vi "Check new DelayFormula and Update DelaysHW.vi"(7 "Update HW?(false)":bool, 8 "error in (no error)":errorcluster, 9 "Delay Formula":string, 10 "ChnlName":string, 11 "BME_DG_System in":refnum<class "BME_DG_System.lvclass">) -> (0 "error out":errorcluster, 2 "Problem Chnls out":string[](array[string]), 3 "BME_DG_System out":refnum<class "BME_DG_System.lvclass">, 4 "Abs. Delay":dbl)   [LabVIEW 2009, in "POLARIS BME DG.lvlib" / "BME_DG_System.lvclass"]
doc: "VIs parses delay formula and calculates new absolute delay value for named channel and all depended channels. If no problems like recursive dependencies and negative absolute delay values are detected the HW will be modified in case if in parameter \"Update HW?\" is true.\n\nATTENTION: in normal case more as one channels have to be modified! Please read online help for BME_DG_Chnl:Parse DelayFormula.vi\n\n\n\nauthor: Alexander Kessler, Helmholtz-Institut-Jena \nmaintainer: Alexander Kessler: alexander.kessler@uni-jena.de\n\nLast Change:\nLicense Agreement for this software:\n\nCopyright (C)\nHelmholtz-Institut-Jena\nFröbelsteg 3\n07743 Jena\nGermany\n\nContact: alexander.kessler@uni-jena.de\n\nThis program is free software; you can redistribute it and/or modify it under the terms of the GNU General Public License as published by the Free Software Foundation; either version 2 of the license, or (at your option) any later version.\n\nThis program is distributed in the hope that it will be useful, but WITHOUT ANY WARRANTY; without even the implied warranty of MERCHANTABILITY or FITNESS FOR A PARTICULAR PURPOSE. See the GNU General License for more details (http://www.gnu.org)."
uses:
  BME_DG_System.lvclass
  BME_DG_Chnl/BME_DG_Chnl.lvclass
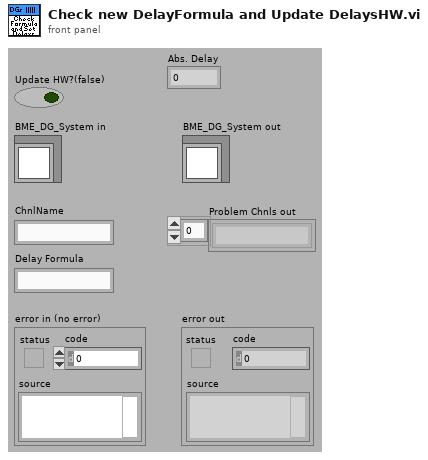
[diagram p1: front panel]
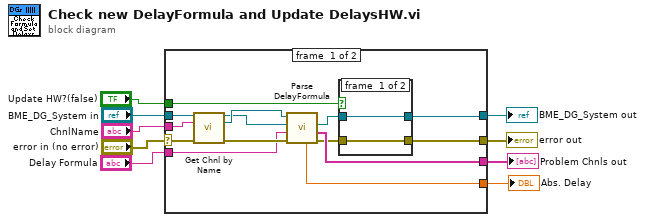
[diagram p0: block diagram]
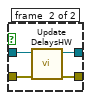
[diagram p2: hidden frame]
diagram:
  n1 = case shown="No Error" "error in (no error)" {
    selector: "error in (no error)" -> [w21 w31]
    tunnel: [w12 w31] -> w8
    tunnel: [w14 w30] -> w6
    tunnel: "BME_DG_System in" -> [w23 w30]
    tunnel: "ChnlName" -> [w22 _]
    tunnel: "Delay Formula" -> [w18 _]
    tunnel: [w16 _] -> w3
    tunnel: "Update HW?(false)" -> [w11 _]
    tunnel: [w10 _] -> w1
    frame #0 {
      n2 = call "Get Chnl by Name.vi"("BME_DG_System in"=w23, "Chnl Name"=w22, "error in (no error)"=w21) -> ("BME_DG_System out"=w17:refnum<class "BME_DG_System.lvclass">, "BME_DG_Chnl"=w20:refnum<class "BME_DG_Chnl.lvclass">, "error out"=w19:errorcluster)  [unwired: 7 in, 3 out]
      n3 = call "Parse DelayFormula.vi"("error in (no error)"=w19, "DelayFormula"=w18, "BME_DG_System"=w17, "BME_DG_Chnl in"=w20) -> ("error out"=w13:errorcluster, "Problem Chnls out"=w16:string[], "BME_DG_System out"=w15:refnum<class "BME_DG_System.lvclass">, "Abs. Delay"=w10:dbl)  [unwired: 4 in]
      n4 = case shown="True" w11 {
        tunnel: w15 -> [w25 w29]
        tunnel: [w25 w28] -> w14
        tunnel: w13 -> [w24 w27]
        tunnel: [w24 w26] -> w12
        frame #0 {
        }
        frame #1 {
          n5 = call "Update DelaysHW.vi"("error in (no error)"=w27, "BME_DG_System in"=w29) -> ("error out"=w26:errorcluster, "BME_DG_System out"=w28:refnum<class "BME_DG_System.lvclass">)  [unwired: 8 in]
        }
      }
    }
    frame #1 {
    }
  }
  "error out" <- w8
  "BME_DG_System out" <- w6
  "Problem Chnls out" <- w3
  "Abs. Delay" <- w1
